vi "AsynchronousScriptName.vi"(10 "data_store_mode":enum16{"Set", "Get"}(ring), 11 "Call Script":string) -> (3 "Call Script":string)   [LabVIEW 2011]
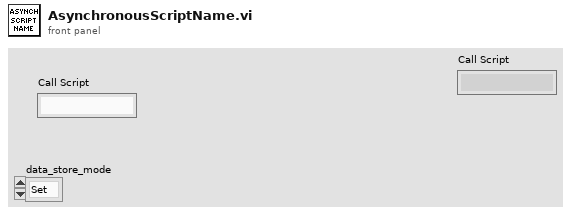
[diagram p1: front panel]
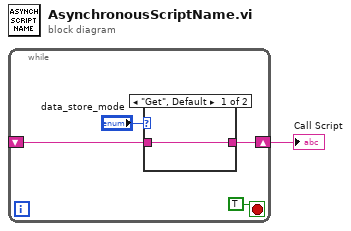
[diagram p0: block diagram]
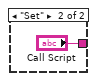
[diagram p2: hidden frame]
diagram:
  n1 = while {
    shift-right: [w3] -> w1
    shift-left: _ -> [w2]
    stop <- TRUE stop-if-true
    n2 = case shown="\"Get\", Default" "data_store_mode" {
      tunnel: [w6 "Call Script"] -> w3
      tunnel: w2 -> [w6 _]
      frame "Get", Default {
      }
      frame "Set" {
      }
    }
  }
  "Call Script" <- w1
